vi "Test Not In Process Loop When Initialized.vi"(8 "error in (no error)":errorcluster, 11 "Test Case In":refnum<class "Process Lifecycle Test.lvclass">) -> (0 "error out":errorcluster, 3 "Test Case Out":refnum<class "Process Lifecycle Test.lvclass">)   [LabVIEW 2020, in "Process Lifecycle Test.lvclass"]
uses:
  Process Lifecycle Test.lvclass
  C:/Program Files (x86)/National Instruments/LabVIEW 2020/vi.lib/Astemes/LUnit/Test Case.lvclass
  source/Framework/Process/Process.lvclass
  source/Framework/Process/Process.lvclass/Process.ctl
  <vilib>/Astemes/LUnit/Test Case.lvclass/Test Case.ctl
  <vilib>/Utility/error.llb/Clear Errors.vi
  <vilib>/Astemes/LUnit/Append Pass Result.vi
  <vilib>/Astemes/LUnit/Append Fail Result.vi
  <vilib>/Astemes/LUnit/Test Case.lvclass
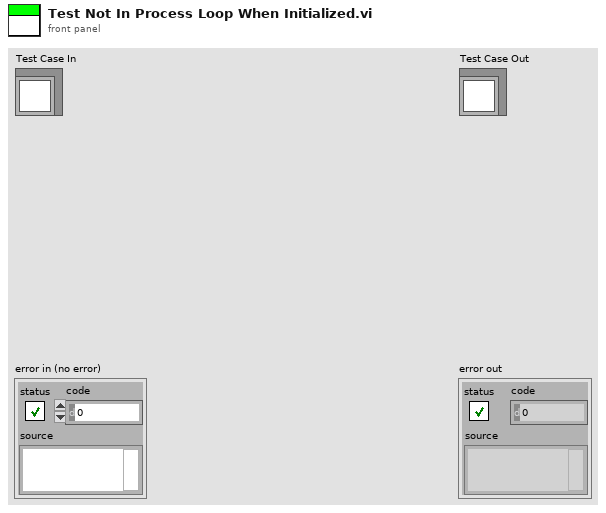
[diagram p1: front panel]
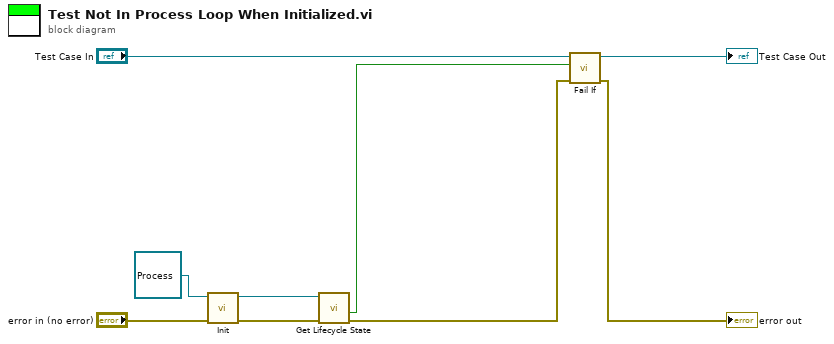
[diagram p0: block diagram]
diagram:
  n1 = call-dynamic "Init.vi"("error in (no error)"="error in (no error)", "Process In"=refnum<class "Process.lvclass"> refnum) -> ("error out"=w3:errorcluster, "Process Out"=w1:refnum<class "Process.lvclass">)  [unwired: 8 in]
  n2 = call "Get Lifecycle State.vi"("error in (no error)"=w3, "Process In"=w1) -> ("error out"=w5:errorcluster, "In Process Loop?"=w4:bool)  [unwired: 6 in, 2 out]
  n3 = call <vilib>:"Fail If.vi"("error in (no error)"=w5, "Fail?"=w4, "LUnit Test Case In"="Test Case In") -> ("error out"=→"error out":errorcluster, "LUnit Test Case Out"=→"Test Case Out":refnum<class "Process Lifecycle Test.lvclass">)  [unwired: 7 in]
